vi "dsf config file property name.vi"() -> (3 "file path property name":string)   [LabVIEW 2020, in "DSF Shared.lvlib"]
uses:
  Shared/DSF Shared.lvlib
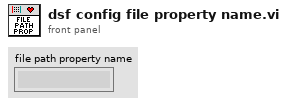
[diagram p1: front panel]
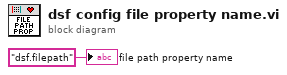
[diagram p0: block diagram]
diagram:
  "file path property name" <- "dsf.filepath" ("Property Name")
